vi "Get Channel UIs.vi"(8 "error in (no error)":errorcluster, 11 "Component UI in":refnum<class "Core Component User Interfaces.lvclass">) -> (0 "error out":errorcluster, 1 "Tx Channel UI":refnum<class "User Interface.lvclass">, 2 "Rx Channel UI":refnum<class "User Interface.lvclass">, 3 "Component UI out":refnum<class "Core Component User Interfaces.lvclass">)   [LabVIEW 2021, in "DSF Core.lvlib" / "Core Component User Interfaces.lvclass"]
uses:
  Core Component User Interfaces.lvclass
  User Interface/User Interface.lvclass
  User Interface/Core/Channel/Core Channel User Interface.lvclass
  C:/dev/git/custom-devices/niveristand-data-sharing-framework-custom-device/Source/Core/Classes/User Interface/User Interface.lvclass
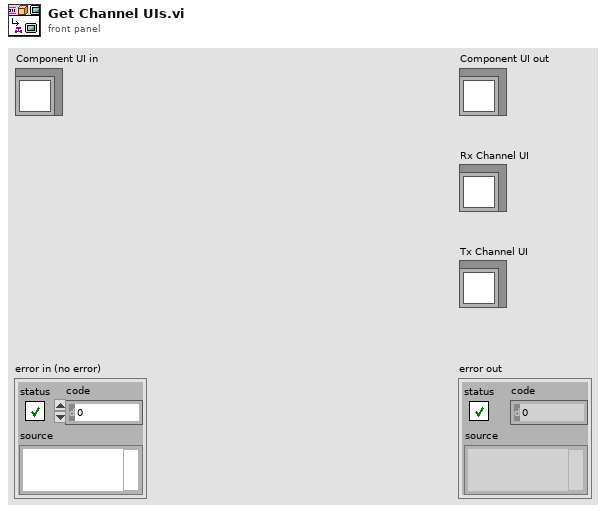
[diagram p1: front panel]
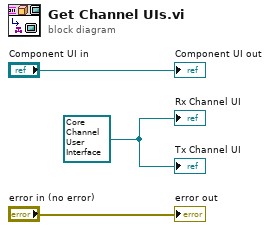
[diagram p0: block diagram]
diagram:
  w1 = refnum<class "Core Channel User Interface.lvclass"> refnum ("DSF Core.lvlib:Core Channel User Interface.lvclass")
  "error out" <- "error in (no error)"
  "Component UI out" <- "Component UI in"
  "Tx Channel UI" <- w1
  "Rx Channel UI" <- w1
